vi "Waveform Attribute, Log to Spreadsheet.vi"(5 "append to file (T)":bool=TRUE, 6 "error in":errorcluster, 7 "delimiter":string=",", 8 "attributes":T1[](array[typedef]) {"Value" format="%#.3f"}, 9 "results file":path=path "C:/Documents and Settings/user/Desktop/Claytons Archive/results.txt") -> (0 "error out":errorcluster, 1 "values":dbl[](array[numeric]) format="%#.3f", 2 "labels":string[](array[string]))   [LabVIEW 2010]
doc: "This function writes all of the waveform attributes to a spreadsheet file."
uses:
  Waveform Attribute Cluster.ctl
  <vilib>/Utility/file.llb/Write To Spreadsheet File (DBL).vi
  <vilib>/Utility/file.llb/Write To Spreadsheet File (string).vi
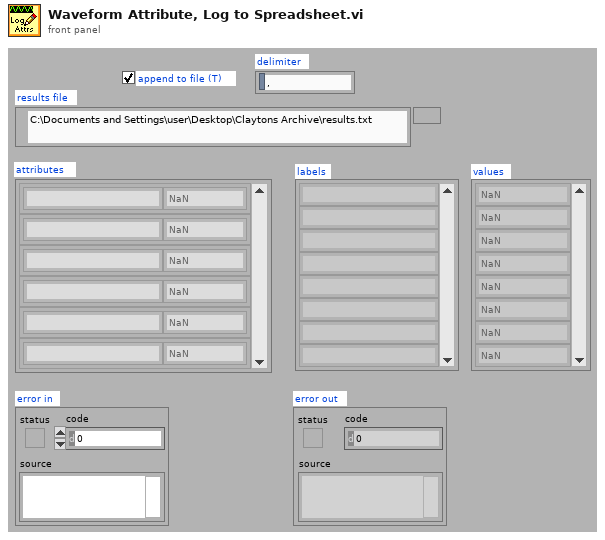
[diagram p1: front panel]
types:
  T1 = typedef "Waveform Attribute Cluster.ctl" = cluster{"Label":string, "Value":dbl}
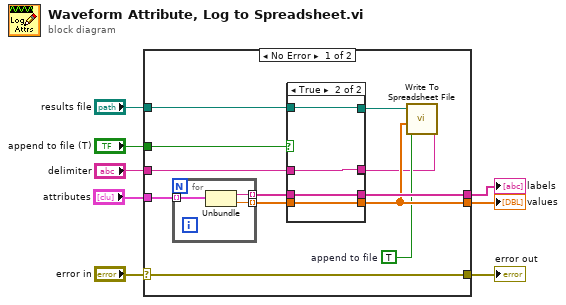
[diagram p0: block diagram]
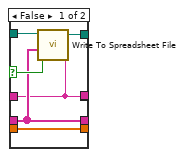
[diagram p2: hidden frame]
diagram:
  n1 = case shown="No Error" "error in" {
    selector: "error in" -> [w18 w34]
    tunnel: [w18 w34] -> w8
    tunnel: "results file" -> [w20 _]
    tunnel: [w12 _] -> w2
    tunnel: "append to file (T)" -> [w15 _]
    tunnel: "attributes" -> [w19 _]
    tunnel: [w13 _] -> w3
    tunnel: "delimiter" -> [w10 _]
    frame No Error {
      w11 = TRUE  # append to file
      n2 = for {
        tunnel: [w33] -> w17 mode=indexing
        tunnel: [w32] -> w14 mode=indexing
        tunnel: w19 -> [w31] mode=indexing
        n3 = Unbundle(w31) -> ("Label"=w33:string, "Value"=w32:dbl)
      }
      n4 = case shown="True" w15 {
        selector: w15 -> [w24 _]
        tunnel: w20 -> [w26 w28]
        tunnel: w17 -> [w23 w30]
        tunnel: [w25 w28] -> w16
        tunnel: w10 -> [w21 w27]
        tunnel: [w23 w30] -> w13
        tunnel: w14 -> [w22 w29]
        tunnel: [w22 w29] -> w12
        tunnel: [w21 w27] -> w9
        tunnel: w10 -> [_ _]
        frame False {
          n5 = call-poly <vilib>:"Write To Spreadsheet File.vi"("delimiter (\\t)"=w21, "append to file? (new file:F)"=w24, "1D data"=w23, "file path (dialog if empty)"=w26) -> ("new file path (Not A Path if cancelled)"=w25:path)  [unwired: 4 in]
        }
        frame True {
        }
      }
      n6 = call-poly <vilib>:"Write To Spreadsheet File.vi"("delimiter (\\t)"=w9, "append to file? (new file:F)"=w11, "1D data"=w12, "file path (dialog if empty)"=w16) -> ()  [unwired: 4 in, 1 out]
    }
    frame Error {
    }
  }
  "error out" <- w8
  "values" <- w2
  "labels" <- w3
